vi "spring - find branch.vi"(8 "error in (no error)":errorcluster, 9 "branch index":i32=-1, 10 "tree data":T1[](array[typedef]), 11 "tag":string) -> (0 "error out":errorcluster, 2 "branch size":i32=-1)   [LabVIEW 2014]
uses:
  spring - node data.ctl
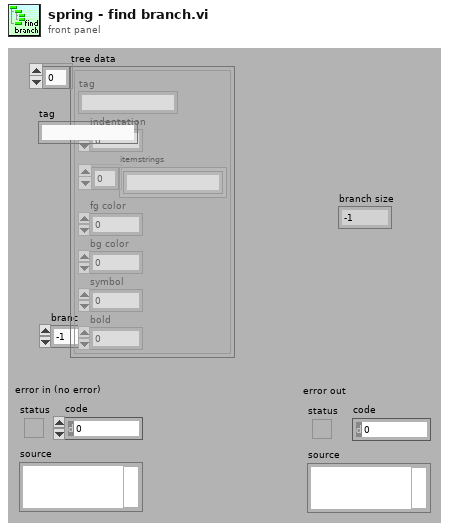
[diagram p1: front panel]
types:
  T1 = typedef "spring - node data.ctl" = cluster{"tag":string, "indentation":i32, "itemstrings":string[], "fg color":u32, "bg color":u32, "symbol":u32, "bold":u32}
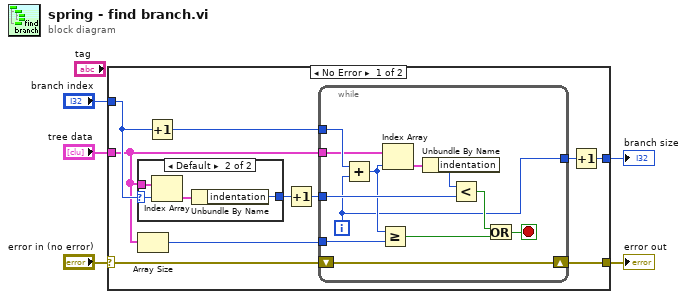
[diagram p0: block diagram]
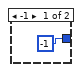
[diagram p2: hidden frame]
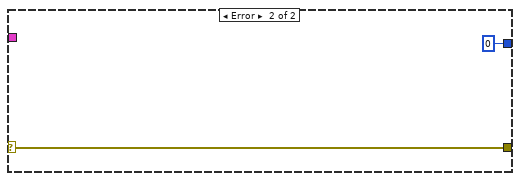
[diagram p3: hidden frame]
diagram:
  n1 = case shown="No Error" "error in (no error)" {
    selector: "error in (no error)" -> [w15 w34]
    tunnel: [w14 w34] -> w5
    tunnel: "tree data" -> [w9 _]
    tunnel: "branch index" -> [w13 _]
    tunnel: [w7 0] -> w2
    frame No Error {
      n2 = case shown="Default" w13 {
        selector: w13 -> [_ w19]
        tunnel: w9 -> [_ w20]
        tunnel: [-1 ("indentation") w17] -> w12
        frame -1 {
        }
        frame Default {
          n3 = Index Array(array=w20, index=w19) -> (element=w18:T1)
          n4 = Unbundle By Name(w18) -> ("indentation"=w17:i32)
        }
      }
      n5 = Array Size(array=w9) -> (size(s)=w6:i32)
      n6 = Increment(x=w13) -> (x+1=w10:i32)
      n7 = Increment(x=w12) -> (x+1=w11:i32)
      n8 = while {
        shift-right: [w29] -> w14
        shift-left: w15 -> [w29]
        tunnel: w9 -> [w30]
        tunnel: w11 -> [w32]
        tunnel: w10 -> [w31]
        tunnel: w6 -> [w26]
        tunnel: [w23] -> w8
        i -> [w23]
        stop <- w27 stop-if-true
        n9 = Add(x=w31, y=w23) -> (x+y=w25:i32)
        n10 = Greater Or Equal?(x=w25, y=w26) -> (x >= y?=w24:bool)
        n11 = Index Array(array=w30, index=w25) -> (element=w21:T1)
        n12 = Unbundle By Name(w21) -> ("indentation"=w22:i32)
        n13 = Less?(x=w22, y=w32) -> (x < y?=w28:bool)
        n14 = Or(x=w28, y=w24) -> (x .or. y?=w27:bool)
      }
      n15 = Increment(x=w8) -> (x+1=w7:i32)
    }
    frame Error {
    }
  }
  "error out" <- w5
  "branch size" <- w2
